vi "Cryo-Con Set PID.vi"(5 "P manual":dbl, 6 "D":dbl, 7 "I":dbl, 8 "Error In":errorcluster, 9 "P":dbl, 10 "Loop number":i32=1, 11 "VISA resource name":refnum<visa-resource-name>) -> (0 "Error Out":errorcluster, 3 "VISA resource name out":refnum<visa-resource-name>)   [LabVIEW 2021]
panel:
  out "resulting string":string
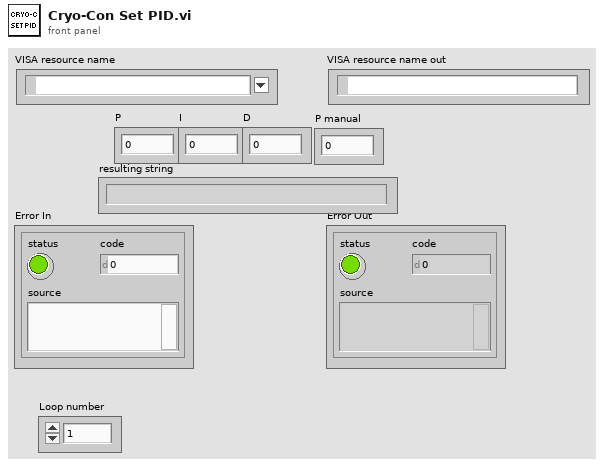
[diagram p1: front panel]
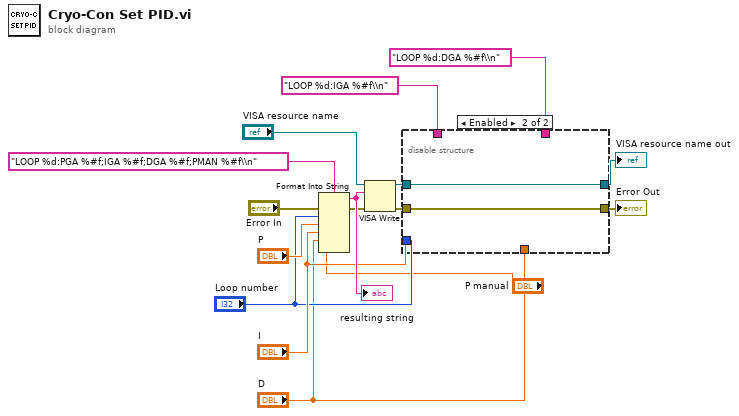
[diagram p0: block diagram]
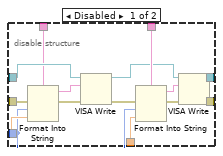
[diagram p2: hidden frame]
diagram:
  n1 = Format Into String(format string="LOOP %d:PGA %#f;IGA %#f;DGA %#f;PMAN %#f\\n", error in="Error In", "Loop number", "P", "I", "D", "P manual") -> (resulting string=w13:string, error out=w12:errorcluster)  [unwired: 1 in]
  "resulting string" <- w13
  n2 = VISA Write(VISA resource name="VISA resource name", write buffer=w13, error in (no error)=w12) -> (VISA resource name out=w10:refnum<visa-resource-name>, error out=w8:errorcluster)  [unwired: 1 out]
  n3 = disable-structure shown="Enabled" {
    disable-tunnel: w10 -> [w31 w33]
    disable-tunnel: "LOOP %d:IGA %#f\\n" ("format string") -> [w30 _]
    disable-tunnel: w8 -> [w29 w32]
    disable-tunnel: "I" -> [w26 _]
    disable-tunnel: "LOOP %d:DGA %#f\\n" ("format string") -> [w25 _]
    disable-tunnel: "Loop number" -> [w24 _]
    disable-tunnel: "D" -> [w23 _]
    disable-tunnel: [w19 w33] -> w3
    disable-tunnel: [w17 w32] -> w2
    frame Disabled {
      n4 = Format Into String(format string=w30, error in=w29, w24, w26) -> (resulting string=w27:string, error out=w28:errorcluster)  [unwired: 1 in]
      n5 = VISA Write(VISA resource name=w31, write buffer=w27, error in (no error)=w28) -> (VISA resource name out=w20:refnum<visa-resource-name>, error out=w22:errorcluster)  [unwired: 1 out]
      n6 = Format Into String(format string=w25, error in=w22, w24, w23) -> (resulting string=w18:string, error out=w21:errorcluster)  [unwired: 1 in]
      n7 = VISA Write(VISA resource name=w20, write buffer=w18, error in (no error)=w21) -> (VISA resource name out=w19:refnum<visa-resource-name>, error out=w17:errorcluster)  [unwired: 1 out]
    }
    frame Enabled {
    }
  }
  "VISA resource name out" <- w3
  "Error Out" <- w2
